vi "Dashboard Main.vi"() -> ()   [LabVIEW 2012]
uses:
  <vilib>/event_ctls.llb/eventvkey.ctl
  <vilib>/Utility/config.llb/Read Key (String).vi
  <vilib>/Utility/config.llb/Read Key (I32).vi
  <vilib>/Utility/config.llb/Write Key (String).vi
  <vilib>/Utility/config.llb/Write Key (I32).vi
  <vilib>/Utility/config.llb/NI_LVConfig.lvlib
panel:
  in  "Camera Settings":T1={"Frate Rate"=30, "Compression"=30, "Size"=1} {"Frate Rate" scale=1.0..30.0; "Size" items=["640x480", "320x240", "160x120"]}
  out "Mode":T2(ring)=enum."Auto Disabled"
  out "Camera IP":string
  in  "Dashboard Tab":T3(tab)
  out "Actual TARF Angle":dbl
  in  "Enable Autonomous":bool=TRUE
  out "Time Left":dbl
  out "Red":bool
  out "Yellow":bool
  out "Green":bool
  out "Tail Closed":bool
  in  "Climber Arm Manual":bool
  out "Climber State":dbl
  out "Actual Climber Arm Position":dbl
  out "Climber Button Unlocked":bool
  out "TARF Down":bool
  in  "Time To Lower TARF In Autonomous":u32=2100
  in  "Time Red":dbl=30.0
  in  "Time Yellow":dbl=50.0
  in  "Climber Arm Tolerance":dbl=0.5
  in  "Dump Speed Inside":dbl=5.0
  in  "Dump Speed Outside":dbl=3.0
  out "TeleOp Elapsed Seconds":dbl
  in  "Autonomous Tarf Angle":dbl=29.0
  in  "Slider":dbl(slide) scale=0.0..100.0 scale format="%#_3g"
  in  "On/Off":bool caption="Solenoid"
  in  "Test Name":u16(ring) items=["Select the test to run...", "Example Test", "-------------------------------", "List of tests is built in robot code.", "Replace with your own automated tests."]
  in  "Test Tree":string(tree)
  in  "Motor":cluster{"Value":dbl, "Enable":bool} {"Value" scale=-1.0..1.0 scale format="%#_3g"}
  out "Progress":T4 {"Test Progress" scale=0.0..100.0}
  in  "Rev/Fwd":cluster{"Forward":bool, "Reverse":bool}
  in  "Ring":u16(ring) items=["Auto", "Fixed indoor", "Fixed outdoor 1", "Fixed outdoor 2", "Fixed fluorescent 1", "Fixed fluorescent 2", "Hold current"]
  in  "Listbox":i32(listbox)
  in  "Viewer":enum32{"Camera Image", "Variables"}(tab)
  out "Mbps":dbl format="%#.1g"
  in  "Enable":bool
  in  "DB Camera Config":bool
  out "Mbps":bool
  out "fps":dbl format="%#.1g"
  out "Image Error Message":string="Timeout in Camera Communications"
  out "Camera Image":T5(plugin-control)
  out "Robot IP":string
  out "Tree":string(tree)
  # "Robot IP:"
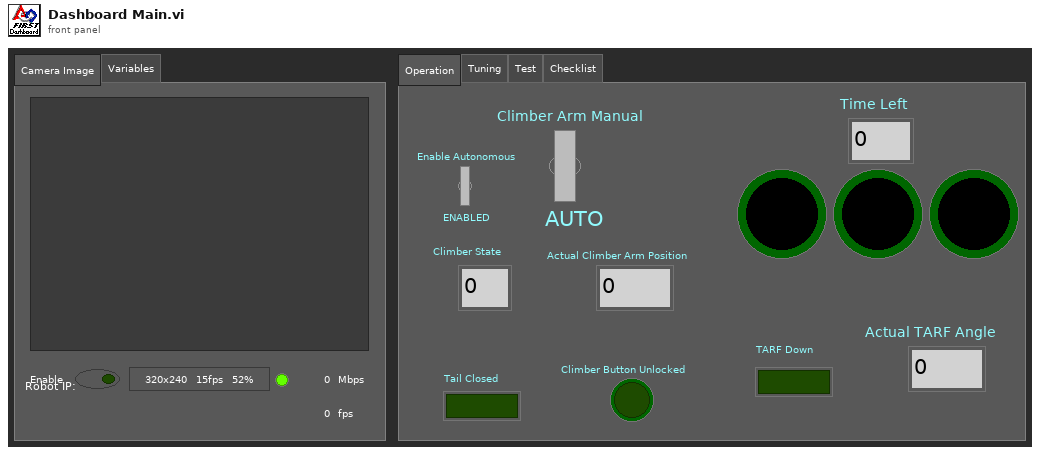
[diagram p1: front panel]
types:
  T1 = cluster{"Frate Rate":i32, "Compression":i32, "Size":u16}
  T2 = enum8{"Tele-Op Disabled", "Tele-Op Enabled", "Auto Disabled", "Auto Enabled", "Test Disabled", "Test Enabled", ""}
  T3 = enum32{"Operation", "Tuning", "Test", "Checklist"}
  T4 = cluster{"Test Progress":u8, "Test Progress Text":string}
  T5 = typedef "IMAQ Image.ctl" = refnum<image>
  T6 = typedef "Image Type" = u32
  T7 = typedef "SkeletonTrackState.ctl" = enum32{"NotTracked", "PositionOnly", "Tracked"}
  T8 = cluster{"TrackingState":u8[], "Position":cluster{"x":sgl, "y":sgl, "z":sgl}, cluster{"x":sgl, "y":sgl, "z":sgl, sgl}[], "TrackState":T7}
  T9 = cluster{cluster{"ScaledToPercentRange":dbl, "ScaledToPercentRange":dbl, "ScaledToPercentRange":dbl}, cluster{bool, bool, bool}}[]
  T10 = cluster{cluster{"ScaledToPercentRange":dbl, "ScaledToPercentRange":dbl, "ScaledToPercentRange":dbl}, cluster{bool, bool, bool}}
  T11 = typedef "LVRectTypeDef.ctl" = cluster{"Left":i16, "Top":i16, "Right":i16, "Bottom":i16}
  T12 = cluster{"Competition mode":bool, "Robot Link":bool, "Autonomous":bool, "Enabled":bool, "E-Stop":bool, "Simulated":bool, "TestMode":bool, "Docked Window":bool}
  T13 = typedef "NI_LVConfig.lvlib/Config Data RefNum.ctl" = refnum<k1>
  T14 = typedef "eventvkey.ctl" = enum16{"ASCII", "Enter", "Return", "Shift", "Ctrl", "Alt", "Cmd", "Opt", "Caps", "NumLock", "Clear", "Break", "Up", "Down", "Left", "Right", "Insert", "Delete", "Home", "End", "PageUp", "PageDown", "Escape", "Help", "Pause", "ScrollLock", "F1", "F2", "F3", "F4", "F5", "F6", "F7", "F8", "F9", "F10", "F11", "F12", "F13", "F14", "F15", "F16", "F17", "F18", "F19", "F20", "F21", "F22", "F23", "F24", "Play", "VolumeUp", "VolumeDown", "Mute", "Two Byte Char"}
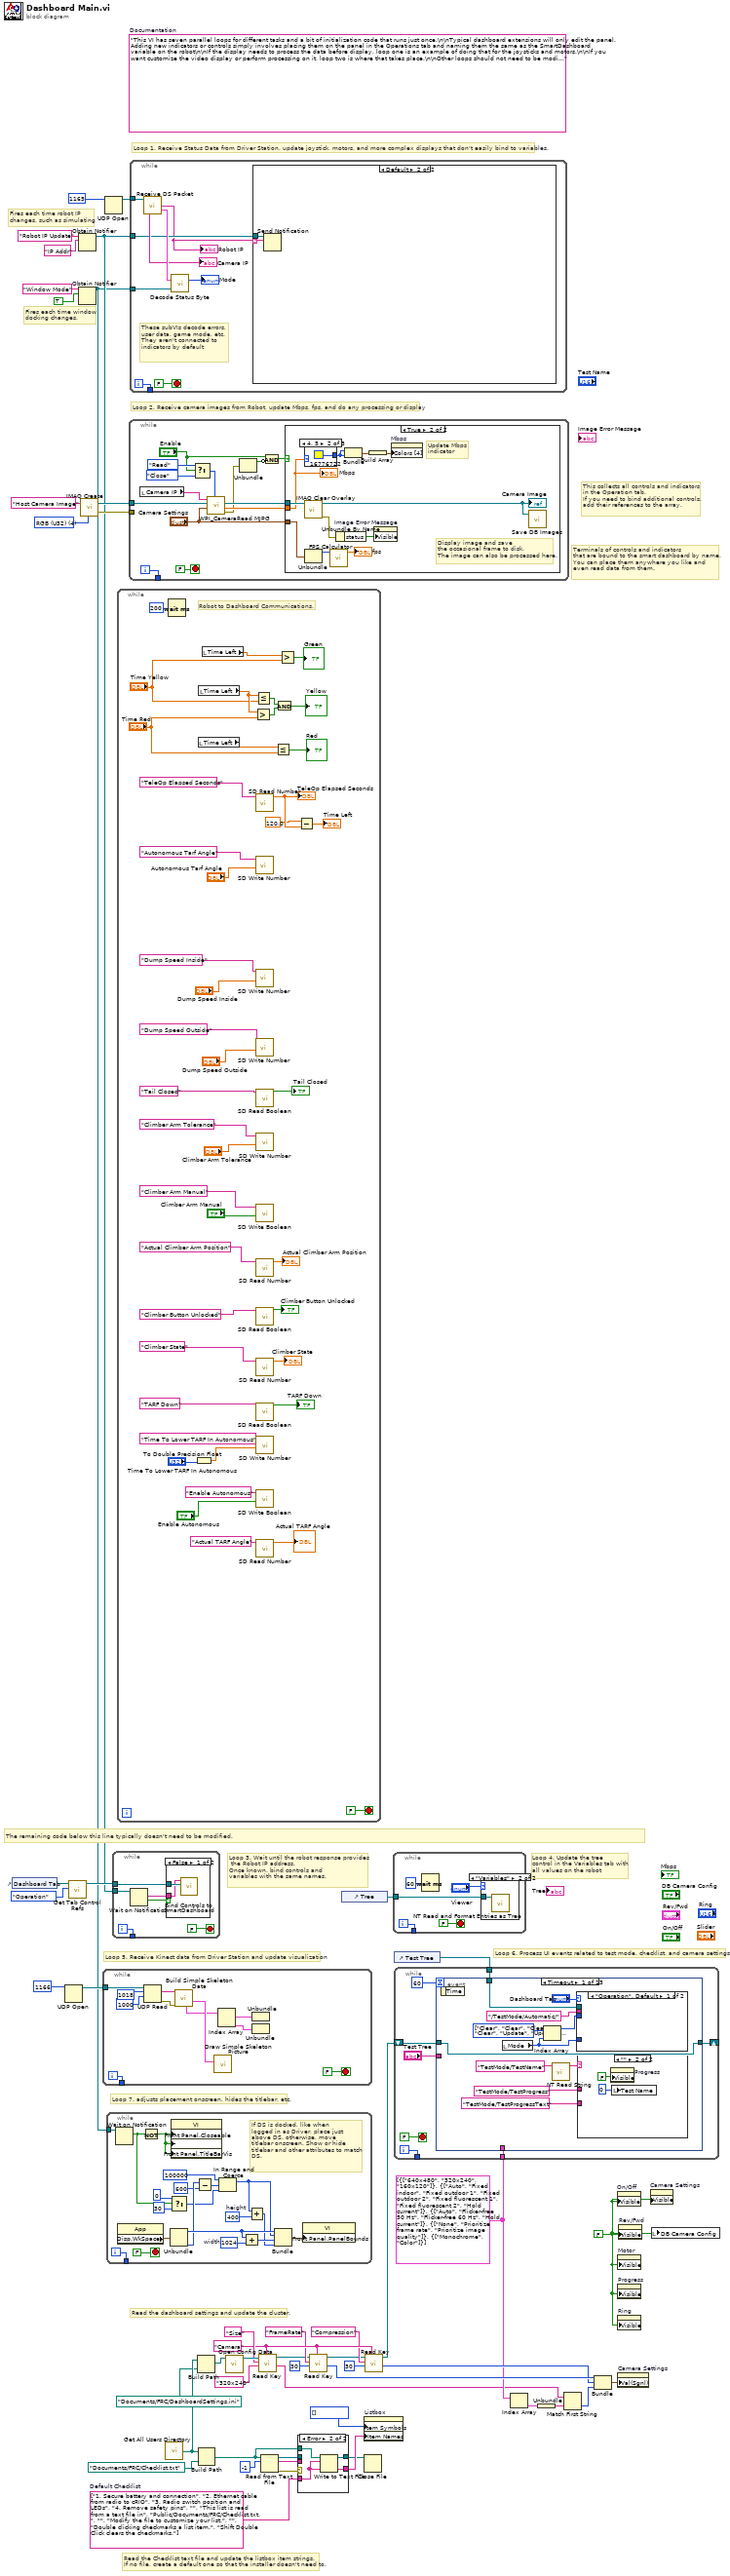
[diagram p0: block diagram]
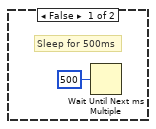
[diagram p3: hidden frame]
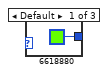
[diagram p4: hidden frame]
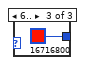
[diagram p5: hidden frame]
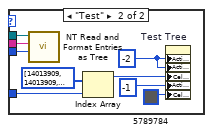
[diagram p7: hidden frame]
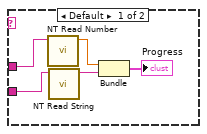
[diagram p8: hidden frame]
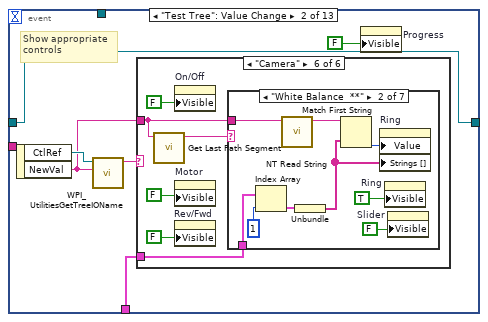
[diagram p9: hidden frame]
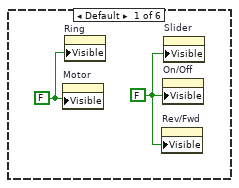
[diagram p10: hidden frame]
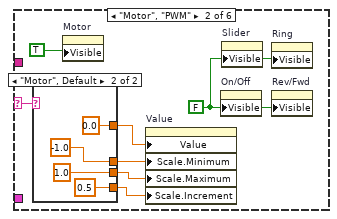
[diagram p11: hidden frame]
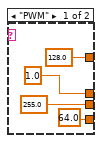
[diagram p12: hidden frame]
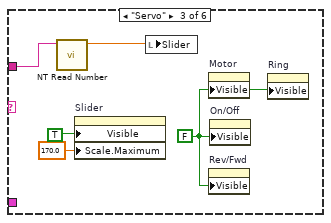
[diagram p13: hidden frame]
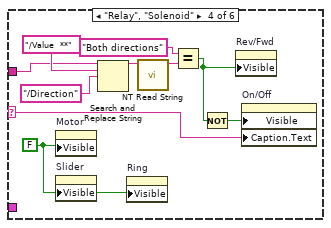
[diagram p14: hidden frame]
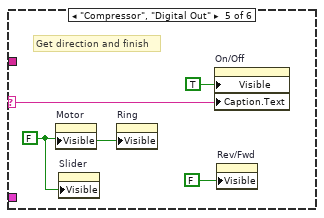
[diagram p15: hidden frame]
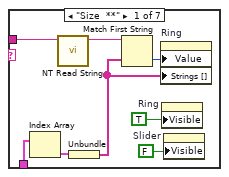
[diagram p16: hidden frame]
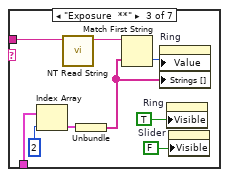
[diagram p17: hidden frame]
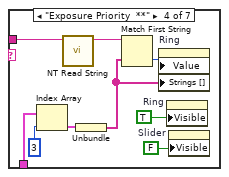
[diagram p18: hidden frame]
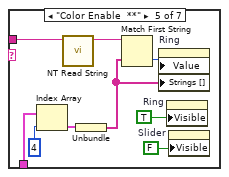
[diagram p19: hidden frame]
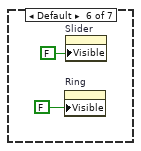
[diagram p20: hidden frame]
diagram:
  w21 = "Camera"
  w13 = cluster{string[]}[] [{["640x480", "320x240", "160x120"]}, {["Auto", "Fixed indoor", "Fixed outdoor 1", "Fixed outdoor 2", "Fixed fluorescent 1", "Fixed fluorescent 2", "Hold current"]}, {["Auto", "Flicker-free 50 Hz", "Flicker-free 60 Hz", "Hold current"]}, {["None", "Prioritize frame rate", "Prioritize image quality"]}, {["Monochrome", "Color"]}]
  w29 = string[] ["1. Secure battery and connection", "2. Ethernet cable from radio to cRIO", "3. Radio switch position and LEDs", "4. Remove safety pins", "", "This list is read from a text file in", "Public/Documents/FRC/Checklist.txt.", "", "Modify the file to customize your list.", "", "Double clicking checkmarks a list item.", "Shift Double Click clears the checkmarks."]  # Default Checklist
  w27 = FALSE ("Visible")
  (unwired) "This VI has seven parallel loops for different tasks and a bit of initialization code that runs just once.\n\nTypical dashboard extensions will only edit the panel. Adding new indicators or controls simply involves placing them on the panel in the Operations tab and naming them the same as the SmartDashboard variable on the robot\n\nIf the display needs to process the data before display, loop one is an example of doing that for the joysticks and motors.\n\nIf you want customize the video display or perform processing on it, loop two is where that takes place.\n\nOther loops should not need to be modified. They are pretty standard, and document the task they perform."  # Documentation
  w50 = T6 4 items=["Grayscale (U8)", "Grayscale (I16)", "Grayscale (SGL)", "Complex (CSG)", "RGB (U32)", "HSL (U32)", "RGB (U64)"] ("Image Type")
  # "Terminals of controls and indicators\nthat are bound to the smart dashboard by name.\nYou can place them anywhere you like and\neven read data from them."
  # "Fires each time robot IP\nchanges, such as simulating"
  # "Fires each time window\ndocking changes."
  # "Read the Checklist text file and update the listbox item strings.\nIf no file, create a default one so that the installer doesn't need to."
  # "This collects all controls and indicators\nin the Operation tab.\nIf you need to bind additional controls,\nadd their references to the array."
  # "The remaining code below this line typically doesn't need to be modified."
  # "Loop 6. Process UI events related to test mode, checklist, and camera settings"
  # "Read the dashboard settings and update the cluster."
  # "Loop 4. Update the tree\ncontrol in the Variables tab with\nall values on the robot"
  # "Loop 3. Wait until the robot response provides\n the Robot IP address.\nOnce known, bind controls and\nvariables with the same names."
  # "Loop 5. Receive Kinect data from Driver Station and update visualization"
  # "Loop 7. adjusts placement onscreen, hides the titlebar, etc."
  # "Loop 1. Receive Status Data from Driver Station, update joystick, motors, and more complex displays that don't easily bind to variables."
  # "Loop 2. Receive camera images from Robot, update Mbps, fps, and do any processing or display"
  n1 = control-ref of="Dashboard Tab"() -> (w43:refnum<vi>)
  n2 = UDP Open(11:u16 1166 ("port")) -> (port=w45:refnum<k16>)  [unwired: 2 in, 4 out]
  n3 = call <vilib>:"Get Tab Control Refs.vi"("Page Index"=enum32{"Operation", "Test"}."Operation" ("Dashboard Tab"), "TabControl in"=w43) -> ("ControlsOnPage"=w44:refnum<vi>[])  [unwired: 9 in]
  n4 = Obtain Notifier(name (unnamed)="Robot IP Update", notification data type="IP Addr" ("name (unnamed)")) -> (notifier out=w40:refnum<notifier>)  [unwired: 2 in, 2 out]
  n5 = Obtain Notifier(name (unnamed)="Window Mode", notification data type=TRUE) -> (notifier out=w33:refnum<notifier>)  [unwired: 2 in, 2 out]
  n6 = call "IMAQ Create"("Image Name"="Host Camera Image", "Image Type"=w50) -> ("New Image"=w48:T5, "error out"=w47:errorcluster)  [unwired: 2 in, 1 out]
  n7 = while {
    tunnel: w45 -> [w61]
    tunnel: [w54] -> _
    i -> [w54]
    stop <- FALSE stop-if-true
    n8 = UDP Read(connection ID=w61, max size (548)=1018 ("bytes to read"), timeout ms (25000)=1000) -> (data out=w59:string, error out=w53:errorcluster)  [unwired: 1 in, 3 out]
    n9 = call "Build Simple Skeleton Data.vi"("error in (no error)"=w53, "data in"=w59) -> ("Skeleton Data"=w60:T8, "Simple Joystick Info"=w57:T9)  [unwired: 5 in, 3 out]
    n10 = call "Draw Simple Skeleton Picture.vi"("Simple Skeleton"=w60) -> ()  [unwired: 10 in, 1 out]
    n11 = Index Array(array=w57) -> (element #1=w56:T10, element #2=w55:T10)  [unwired: 2 in]
    n12 = Unbundle(w56) -> ()  [unwired: 2 out]
    n13 = Unbundle(w55) -> ()  [unwired: 2 out]
  }
  n14 = UDP Open(11:u16 1165 ("port")) -> (port=w51:refnum<k16>)  [unwired: 2 in, 4 out]
  n15 = while {
    tunnel: w33 -> [w82]
    tunnel: [w80] -> _
    i -> [w80]
    stop <- FALSE stop-if-true
    w72 = 1024  # width
    w75 = 400  # height
    # "If DS is docked, like when\nlogged in as Driver, place just\nabove DS, otherwise, move\ntitlebar onscreen. Show or hide\ntitlebar and other attributes to match\nDS."
    n16 = Wait on Notification(notifier=w82) -> (notification=w67:bool)  [unwired: 3 in, 3 out]
    n17 = property class="App"() -> ("Disp.WkSpace"=w78:T11)  [unwired: 2 in, 2 out]
    n18 = Not(x=w67) -> (.not. x?=w81:bool)
    n19 = Unbundle(w78) -> ("Left"=w76:i16, "Bottom"=w73:i16)  [unwired: 2 out]
    n20 = Select(t=0, s=w67, f=30) -> (s? t:f=w66:i32)
    n21 = property class="VI"("Front Panel.Closeable"=w81, "Front Panel.Minimizeable"=w81, "Front Panel.TitleBarVis"=w81) -> ()  [unwired: 2 in, 2 out]
    n22 = Subtract(x=w73, y=600) -> (x-y=w70:i32)
    n23 = In Range and Coerce(upper limit=100000, x=w70, lower limit=w66) -> (coerced(x)=w64:i32)  [unwired: 1 out]
    n24 = Add(x=w76, y=w72) -> (x+y=w77:i32)
    n25 = Add(x=w64, y=w75) -> (x+y=w74:i32)
    n26 = Bundle("Left"=w76, w64, w77, w74) -> (w79:cluster{"Left":i16, i32, i32, i32})  [unwired: 1 out]
    n27 = property class="VI"("Front Panel.PanelBounds"=w79) -> ()  [unwired: 2 in, 2 out]
  }
  n28 = while {
    tunnel: w44 -> [w89]
    tunnel: w40 -> [w86]
    tunnel: [w84] -> _
    i -> [w84]
    stop <- FALSE stop-if-true
    n29 = Wait on Notification(notifier=w86) -> (notification=w85:string, timed out?=w87:bool)  [unwired: 3 in, 2 out]
    n30 = case shown="False" w87 {
      tunnel: w89 -> [w91 _]
      tunnel: w85 -> [w90 _]
      frame False {
        n31 = call <vilib>:"Bind Controls to SmartDashboard.vi"("Bound Control Refs"=w91, "Server IP Address"=w90) -> ()  [unwired: 10 in]
      }
      frame True {
      }
    }
  }
  n32 = while {
    stop <- FALSE stop-if-true
    # "Robot to Dashboard Communications."
    n33 = Wait (ms)(milliseconds to wait=u32 200) -> ()  [unwired: 1 out]
    n34 = To Double Precision Float(number="Time To Lower TARF In Autonomous") -> (double precision float=w104:dbl)
    n35 = local read "Time Left"() -> (w115:dbl)
    n36 = local read "Time Left"() -> (w119:dbl)
    n37 = local read "Time Left"() -> (w121:dbl)
    n38 = Greater?(x=w119, y="Time Red") -> (0:w117:bool)
    n39 = Less Or Equal?(x=w119, y="Time Yellow") -> (x <= y?=w118:bool)
    n40 = call <vilib>:"SD Read Number.vi"("Name"="TeleOp Elapsed Seconds") -> ("Numeric"=w112:dbl)  [unwired: 8 in, 2 out]
    "TeleOp Elapsed Seconds" <- w112
    n41 = call <vilib>:"SD Write Number.vi"("Numeric"="Autonomous Tarf Angle", "Name"="Autonomous Tarf Angle") -> ()  [unwired: 8 in, 2 out]
    n42 = call <vilib>:"SD Write Number.vi"("Numeric"="Dump Speed Inside", "Name"="Dump Speed Inside") -> ()  [unwired: 8 in, 2 out]
    n43 = call <vilib>:"SD Write Number.vi"("Numeric"="Dump Speed Outside", "Name"="Dump Speed Outside") -> ()  [unwired: 8 in, 2 out]
    n44 = call <vilib>:"SD Read Boolean.vi"("Name"="Tail Closed") -> ("Boolean"=→"Tail Closed":bool)  [unwired: 8 in, 2 out]
    n45 = call <vilib>:"SD Write Number.vi"("Numeric"="Climber Arm Tolerance", "Name"="Climber Arm Tolerance") -> ()  [unwired: 8 in, 2 out]
    n46 = call <vilib>:"SD Write Boolean.vi"("Boolean"="Climber Arm Manual", "Name"="Climber Arm Manual") -> ()  [unwired: 8 in, 2 out]
    n47 = call <vilib>:"SD Read Number.vi"("Name"="Actual Climber Arm Position") -> ("Numeric"=→"Actual Climber Arm Position":dbl)  [unwired: 8 in, 2 out]
    n48 = call <vilib>:"SD Read Boolean.vi"("Name"="Climber Button Unlocked") -> ("Boolean"=→"Climber Button Unlocked":bool)  [unwired: 8 in, 2 out]
    n49 = call <vilib>:"SD Read Number.vi"("Name"="Climber State") -> ("Numeric"=→"Climber State":dbl)  [unwired: 8 in, 2 out]
    n50 = call <vilib>:"SD Read Boolean.vi"("Name"="TARF Down") -> ("Boolean"=→"TARF Down":bool)  [unwired: 8 in, 2 out]
    n51 = call <vilib>:"SD Write Number.vi"("Numeric"=w104, "Name"="Time To Lower TARF In Autonomous") -> ()  [unwired: 8 in, 2 out]
    n52 = call <vilib>:"SD Write Boolean.vi"("Boolean"="Enable Autonomous", "Name"="Enable Autonomous") -> ()  [unwired: 8 in, 2 out]
    n53 = call <vilib>:"SD Read Number.vi"("Name"="Actual TARF Angle") -> ("Numeric"=→"Actual TARF Angle":dbl)  [unwired: 8 in, 2 out]
    n54 = Less Or Equal?(x=w115, y="Time Red") -> (x <= y?=→"Red":bool)
    n55 = And(x=w118, y=w117) -> (x .and. y?=→"Yellow":bool)
    n56 = Greater?(x=w121, y="Time Yellow") -> (0:→"Green":bool)
    n57 = Subtract(x=120.0, y=w112) -> (x-y=→"Time Left":dbl)
  }
  n58 = while {
    tunnel: w48 -> [w144]
    tunnel: w47 -> [_]
    tunnel: [w147] -> _
    i -> [w147]
    stop <- FALSE stop-if-true
    n59 = local read "Camera IP"() -> (w146:string)
    n60 = Select(t=enum16{"Read", "Reopen", "Close"}."Read" ("Operation"), s="Enable", f=enum16{"Read", "Reopen", "Close"}."Close" ("Operation")) -> (s? t:f=w139:enum16{"Read", "Reopen", "Close"})
    n61 = call <vilib>:"WPI_CameraRead MJPG.vi"("Operation"=w139, "Camera Settings"="Camera Settings", "Image"=w144, "address"=w146) -> ("error out"=w138:errorcluster, "Bandwidth (kbps)"=w142:dbl, "Image Out"=w143:T5)  [unwired: 5 in]
    n62 = Unbundle(w138) -> ("status"=w136:bool)  [unwired: 2 out]
    n63 = Compound Arithmetic op=AND("Enable", invert w136) -> (w135:bool)
    n64 = case shown="True" w135 {
      tunnel: "Camera Settings" -> [_ w151]
      tunnel: w143 -> [_ w154]
      tunnel: w142 -> [_ w153]
      frame False {
        # "Sleep for 500ms"
        n65 = Wait Until Next ms Multiple(millisecond multiple=u32 500) -> ()  [unwired: 1 out]
      }
      frame True {
        # "Display image and save\nthe occasional frame to disk.\nThe image can also be processed here."
        # "Update Mbps\nindicator"
        n66 = call "IMAQ Clear Overlay"("Image"=w154) -> ("error out"=w159:errorcluster, "Image Out"=w158:T5)  [unwired: 2 in, 7 out]
        "Camera Image" <- w158
        n67 = case shown="4, 5" w153 {
          tunnel: [u32 6618880 ("Color Box") u32 16776722 ("Color Box") u32 16716800 ("Color Box")] -> w155
          frame Default {
          }
          frame 4, 5 {
          }
          frame 6.. {
          }
        }
        n68 = Unbundle(w151) -> ("Frate Rate"=w150:i32)  [unwired: 2 out]
        n69 = call "FPS Calculator.vi"("Average Count"=w150) -> ("fps"=→"fps":dbl)  [unwired: 10 in]
        n70 = Unbundle By Name(w159) -> ("status"=w160:bool)
        n71 = Bundle("Color Box"=w155, "Color Box"=w155) -> (w157:cluster{"Color Box":u32, "Color Box":u32})  [unwired: 1 out]
        n72 = Build Array(w157) -> (w156:cluster{"Color Box":u32, "Color Box":u32}[])
        n73 = property on="Image Error Message" class="Str"("Visible"=w160) -> ()  [unwired: 2 in, 2 out]
        n74 = property on="Mbps" class="Bool (strict)"("Colors [4]"=w156) -> ()  [unwired: 2 in, 2 out]
        n75 = call "Save DB Images.vi"("Image"=w158) -> ()  [unwired: 2 in, 1 out]
        "Mbps" <- w153
      }
    }
  }
  n76 = while {
    tunnel: w51 -> [w170]
    tunnel: w40 -> [w165]
    tunnel: w33 -> [w169]
    tunnel: [w166] -> _
    i -> [w166]
    stop <- FALSE stop-if-true
    # "These subVIs decode errors, user data, game mode, etc.\nThey aren't connected to indicators by default"
    n77 = call "Receive DS Packet.vi"("Recv Socket"=w170) -> ("Robot IP Address"=w164:string, "Status"=w171:T12, "Camera IP Address"=→"Camera IP":string)  [unwired: 1 in, 11 out]
    "Robot IP" <- w164
    n78 = call "Decode Status Byte.vi"("Window Mode Notifier"=w169, "Status"=w171) -> ("Mode"=→"Mode":T2)  [unwired: 1 out]
    n79 = case shown="Default" w164 {
      selector: w164 -> [_ w173]
      tunnel: w165 -> [_ w174]
      frame "0.0.0.0" {
        # "Robot not responding, don't poll the variables"
      }
      frame Default {
        n80 = Send Notification(notification=w173, notifier=w174) -> ()  [unwired: 1 in, 2 out]
      }
    }
  }
  n81 = call "Get All Users Directory.vi"() -> ("All User Path"=w26:path)
  n82 = Build Path(base path=w26, name or relative path=path "Documents/FRC/DashboardSettings.ini") -> (appended path=w25:path)
  n83 = Build Path(base path=w26, name or relative path=path "Documents/FRC/Checklist.txt") -> (appended path=w30:path)
  n84 = call <vilib>:"Open Config Data.vi"("configuration file path"=w25) -> ("refnum"=w24:T13)  [unwired: 8 in, 2 out]
  n85 = call-poly <vilib>:"Read Key.vi"("section"=w21, "default value"="320x240", "key"="Size", "refnum"=w24) -> ("value"=w11:string, "refnum out"=w6:T13)  [unwired: 2 in, 4 out]
  n86 = Read from Text File(file (use dialog)=w30, count=-1 ("timeout ms (25000)")) -> (refnum out=w8:refnum<file>, text=w31:string[], error out=w32:errorcluster)  [unwired: 2 in, 1 out]
  n87 = case shown="Error" w32 {
    tunnel: w31 -> [w176 _]
    tunnel: [w176 w178] -> w28
    tunnel: w29 -> [_ w178]
    tunnel: w30 -> [_ w179]
    tunnel: [w175 w177] -> w7
    tunnel: w8 -> [w175 _]
    frame No Error {
    }
    frame Error {
      n88 = Write to Text File(file (use dialog)=w179, text=w178) -> (refnum out=w177:refnum<file>)  [unwired: 2 in, 2 out]
    }
  }
  n89 = call-poly <vilib>:"Read Key.vi"("section"=w21, "default value"=30, "key"="FrameRate", "refnum"=w6) -> ("value"=w16:i32, "refnum out"=w5:T13)  [unwired: 1 in, 5 out]
  n90 = control-ref of="Tree"() -> (w2:refnum<vi>)
  n91 = property on="Listbox" class="LstBox (strict)"("Item Symbols"=i32[] [], "Item Names"=w28) -> ()  [unwired: 2 in, 2 out]
  n92 = Close File(refnum=w7) -> ()  [unwired: 1 in, 2 out]
  n93 = call-poly <vilib>:"Read Key.vi"("section"=w21, "default value"=30, "key"="Compression", "refnum"=w5) -> ("value"=w15:i32, "refnum out"=w3:T13)  [unwired: 1 in, 5 out]
  n94 = while {
    tunnel: [w181] -> _
    tunnel: w2 -> [w180]
    i -> [w181]
    stop <- FALSE stop-if-true
    n95 = Wait (ms)(milliseconds to wait=u32 60) -> ()  [unwired: 1 out]
    n96 = case shown="\"Variables\"" "Viewer" {
      tunnel: w180 -> [_ w185]
      frame Default {
      }
      frame "Variables" {
        n97 = call <vilib>:"NT Read and Format Entries as Tree.vi"("Tree Refnum"=w185) -> ()  [unwired: 9 in, 2 out]
      }
    }
  }
  n98 = control-ref of="Test Tree"() -> (w1:refnum<vi>)
  n99 = while {
    tunnel: w13 -> [w190]
    shift-right: [w189] -> _
    shift-left: w3 -> [w188]
    tunnel: [w187] -> _
    tunnel: w1 -> [w186]
    i -> [w187]
    stop <- FALSE stop-if-true
    n100 = event shown="[0] Timeout" {
      selector: _ -> [_ _ _ _ _ _ _ _ _ _ _ _ _]
      dyn-events: _ -> [_ _ _ _ _ _ _ _ _ _ _ _ _]
      timeout: u32 60 ("milliseconds to wait") -> [_ _ _ _ _ _ _ _ _ _ _ _ _]
      tunnel: w186 -> [w200 _ _ _ _ _ _ _ _ _ _ _ _]
      tunnel: "Test Tree" -> [_ _ _ _ _ _ _ _ w394 w402 w404 w408 w416]
      tunnel: w190 -> [_ w222 _ _ _ _ w358 w388 _ _ _ _ _]
      tunnel: [w194 w221 _ w324 w332 w344 w357 w381 w393 w400 w403 w407 w415] -> w189
      tunnel: w188 -> [w194 w221 _ w324 w332 w344 w356 w381 w393 w400 w403 w407 w415]
      event Timeout {
        w199 = enum16{"Update", "Clear"}[] [enum."Clear", enum."Clear", enum."Clear", enum."Clear", enum."Update", enum."Update", enum."Clear"] items=["Update", "Clear"]
        n101 = event-data() -> ()  [unwired: 1 in, 1 out]
        n102 = local read "Mode"() -> (w197:T2)
        n103 = Index Array(array=w199, index=w197) -> (element=w198:enum16{"Update", "Clear"})
        n104 = call <vilib>:"NT Read String.vi"("Name"="TestMode/TestName") -> ("String"=w203:string)  [unwired: 9 in, 1 out]
        n105 = case shown="\"Operation\", Default" "Dashboard Tab" {
          tunnel: w200 -> [_ w213]
          tunnel: "/TestMode/Automatic/" ("Name Pattern") -> [_ w212]
          tunnel: w198 -> [_ w211]
          tunnel: w197 -> [_ w209]
          frame "Operation", Default {
          }
          frame "Test" {
            w208 = -2 ("Active Item:Row Number")
            n106 = call <vilib>:"NT Read and Format Entries as Tree.vi"("Operation"=w211, "Name Pattern"=w212, "Tree Refnum"=w213) -> ()  [unwired: 7 in, 2 out]
            n107 = Index Array(array=u32[] [14013909, 14013909, 14013909, 14013909, 14013909, 16777215, 14013909], index=w209) -> (element=w207:u32)
            n108 = property on="Test Tree" class="Tree (strict)"("Active Item Row Number"=w208, "ActiveColNum"=w208, "CellBG"=w207, "Active Item Row Number"=-1 ("Active Item:Row Number"), "CellBG"=u32 5789784 ("Color Box")) -> ()  [unwired: 2 in, 2 out]
          }
        }
        n109 = case shown="\"\"" w203 {
          tunnel: "TestMode/TestProgress" ("Name") -> [w215 _]
          tunnel: "TestMode/TestProgressText" ("Name") -> [w214 _]
          frame Default {
            n110 = call <vilib>:"NT Read Number.vi"("Name"=w215) -> ("Numeric"=w216:dbl)  [unwired: 9 in, 1 out]
            n111 = call <vilib>:"NT Read String.vi"("Name"=w214) -> ("String"=w217:string)  [unwired: 9 in, 1 out]
            n112 = Bundle("Numeric"=w216, "String"=w217) -> (→"Progress":cluster{"Numeric":dbl, "String":string})  [unwired: 1 in]
          }
          frame "" {
            n113 = property on="Progress" class="Clust (strict)"("Visible"=FALSE) -> ()  [unwired: 2 in, 2 out]
            n114 = local write "Test Name"(u16 0) -> ()
          }
        }
      }
      event "Test Tree": Value Change {
        # "Show appropriate\ncontrols"
        n115 = event-data() -> ("CtlRef"=w225:refnum<vi>, "NewVal"=w223:string)  [unwired: 1 in]
        n116 = call <vilib>:"WPI_UtilitiesGetTreeIOName.vi"("NewVal"=w223, "TreeControl in"=w225) -> ("I/O Name"=w226:string)  [unwired: 9 in]
        n117 = case shown="\"Camera\"" w226 {
          selector: w226 -> [_ w233 _ w251 w260 _]
          tunnel: w223 -> [_ _ w248 w250 _ w267]
          tunnel: w222 -> [_ _ _ _ _ w266]
          frame Default {
            w228 = FALSE ("Visible")
            w227 = FALSE ("Visible")
            n118 = property on="Motor" class="Clust (strict)"("Visible"=w227) -> ()  [unwired: 2 in, 2 out]
            n119 = property on="Ring" class="Ring (strict)"("Visible"=w227) -> ()  [unwired: 2 in, 2 out]
            n120 = property on="Rev/Fwd" class="Clust (strict)"("Visible"=w228) -> ()  [unwired: 2 in, 2 out]
            n121 = property on="On/Off" class="Bool (strict)"("Visible"=w228) -> ()  [unwired: 2 in, 2 out]
            n122 = property on="Slider" class="Slide (strict)"("Visible"=w228) -> ()  [unwired: 2 in, 2 out]
          }
          frame "Motor", "PWM" {
            w234 = FALSE ("Visible")
            n123 = case shown="\"Motor\", Default" w233 {
              tunnel: [1.0 ("Value") -1.0 ("Value")] -> w232
              tunnel: [255.0 ("Value") 1.0 ("Value")] -> w231
              tunnel: [128.0 ("Value") 0.0 ("Value")] -> w230
              tunnel: [64.0 ("Value") 0.5 ("Value")] -> w229
              frame "PWM" {
              }
              frame "Motor", Default {
              }
            }
            n124 = property on="Motor" class="Clust (strict)"("Visible"=TRUE) -> ()  [unwired: 2 in, 2 out]
            n125 = property on="Value" class="Slide (strict)"("Value"=w230, "Scale.Minimum"=w232, "Scale.Maximum"=w231, "Scale.Increment"=w229) -> ()  [unwired: 2 in, 2 out]
            n126 = property on="On/Off" class="Bool (strict)"("Visible"=w234) -> ()  [unwired: 2 in, 2 out]
            n127 = property on="Slider" class="Slide (strict)"("Visible"=w234) -> ()  [unwired: 2 in, 2 out]
            n128 = property on="Ring" class="Ring (strict)"("Visible"=w234) -> ()  [unwired: 2 in, 2 out]
            n129 = property on="Rev/Fwd" class="Clust (strict)"("Visible"=w234) -> ()  [unwired: 2 in, 2 out]
          }
          frame "Servo" {
            w246 = FALSE ("Visible")
            n130 = call <vilib>:"NT Read Number.vi"("Name"=w248) -> ("Numeric"=w247:dbl)  [unwired: 9 in, 1 out]
            n131 = property on="Slider" class="Slide (strict)"("Visible"=TRUE, "Scale.Maximum"=170.0 ("Scale.Range:Maximum")) -> ()  [unwired: 2 in, 2 out]
            n132 = local write "Slider"(w247) -> ()
            n133 = property on="Motor" class="Clust (strict)"("Visible"=w246) -> ()  [unwired: 2 in, 2 out]
            n134 = property on="Rev/Fwd" class="Clust (strict)"("Visible"=w246) -> ()  [unwired: 2 in, 2 out]
            n135 = property on="On/Off" class="Bool (strict)"("Visible"=w246) -> ()  [unwired: 2 in, 2 out]
            n136 = property on="Ring" class="Ring (strict)"("Visible"=w246) -> ()  [unwired: 2 in, 2 out]
          }
          frame "Relay", "Solenoid" {
            w249 = FALSE ("Visible")
            n137 = property on="Motor" class="Clust (strict)"("Visible"=w249) -> ()  [unwired: 2 in, 2 out]
            n138 = property on="Slider" class="Slide (strict)"("Visible"=w249) -> ()  [unwired: 2 in, 2 out]
            n139 = Search and Replace String(input string=w250, search string="/Value  **", replace string="/Direction") -> (result string=w256:string)  [unwired: 5 in, 3 out]
            n140 = property on="Ring" class="Ring (strict)"("Visible"=w249) -> ()  [unwired: 2 in, 2 out]
            n141 = call <vilib>:"NT Read String.vi"("Name"=w256) -> ("String"=w254:string)  [unwired: 9 in, 1 out]
            n142 = Equal?(x="Both directions", y=w254) -> (x = y?=w252:bool)
            n143 = Not(x=w252) -> (.not. x?=w253:bool)
            n144 = property on="Rev/Fwd" class="Clust (strict)"("Visible"=w252) -> ()  [unwired: 2 in, 2 out]
            n145 = property on="On/Off" class="Bool (strict)"("Visible"=w253, "Caption.Text"=w251) -> ()  [unwired: 2 in, 2 out]
          }
          frame "Compressor", "Digital Out" {
            w259 = FALSE ("Visible")
            # "Get direction and finish"
            n146 = property on="Motor" class="Clust (strict)"("Visible"=w259) -> ()  [unwired: 2 in, 2 out]
            n147 = property on="Slider" class="Slide (strict)"("Visible"=w259) -> ()  [unwired: 2 in, 2 out]
            n148 = property on="Ring" class="Ring (strict)"("Visible"=w259) -> ()  [unwired: 2 in, 2 out]
            n149 = property on="On/Off" class="Bool (strict)"("Visible"=TRUE, "Caption.Text"=w260) -> ()  [unwired: 2 in, 2 out]
            n150 = property on="Rev/Fwd" class="Clust (strict)"("Visible"=FALSE) -> ()  [unwired: 2 in, 2 out]
          }
          frame "Camera" {
            n151 = call <vilib>:"Get Last Path Segment.vi"("String in"=w267) -> ("String out"=w268:string)  [unwired: 10 in]
            n152 = property on="On/Off" class="Bool (strict)"("Visible"=FALSE) -> ()  [unwired: 2 in, 2 out]
            n153 = property on="Motor" class="Clust (strict)"("Visible"=FALSE) -> ()  [unwired: 2 in, 2 out]
            n154 = property on="Rev/Fwd" class="Clust (strict)"("Visible"=FALSE) -> ()  [unwired: 2 in, 2 out]
            n155 = case shown="\"White Balance  **\"" w268 {
              tunnel: w267 -> [w274 w283 w292 w301 w310 _ w316]
              tunnel: w266 -> [w272 w280 w289 w298 w307 _ _]
              frame "Size  **" {
                n156 = Index Array(array=w272) -> (element=w271:cluster{string[]})  [unwired: 1 in]
                n157 = call <vilib>:"NT Read String.vi"("Name"=w274) -> ("String"=w273:string)  [unwired: 9 in, 1 out]
                n158 = Unbundle(w271) -> (w269:string[])
                n159 = Match First String(2:w269, 3:w273) -> (0:w270:i32)  [unwired: 1 out]
                n160 = property on="Ring" class="Ring (strict)"("Value"=w270, "Strings []"=w269) -> ()  [unwired: 2 in, 2 out]
                n161 = property on="Ring" class="Ring (strict)"("Visible"=TRUE) -> ()  [unwired: 2 in, 2 out]
                n162 = property on="Slider" class="Slide (strict)"("Visible"=FALSE) -> ()  [unwired: 2 in, 2 out]
              }
              frame "White Balance  **" {
                n163 = Index Array(array=w280, index=1) -> (element=w281:cluster{string[]})
                n164 = call <vilib>:"NT Read String.vi"("Name"=w283) -> ("String"=w282:string)  [unwired: 9 in, 1 out]
                n165 = Unbundle(w281) -> (w278:string[])
                n166 = Match First String(2:w278, 3:w282) -> (0:w277:i32)  [unwired: 1 out]
                n167 = property on="Ring" class="Ring (strict)"("Value"=w277, "Strings []"=w278) -> ()  [unwired: 2 in, 2 out]
                n168 = property on="Ring" class="Ring (strict)"("Visible"=TRUE) -> ()  [unwired: 2 in, 2 out]
                n169 = property on="Slider" class="Slide (strict)"("Visible"=FALSE) -> ()  [unwired: 2 in, 2 out]
              }
              frame "Exposure  **" {
                n170 = Index Array(array=w289, index=2) -> (element=w290:cluster{string[]})
                n171 = call <vilib>:"NT Read String.vi"("Name"=w292) -> ("String"=w291:string)  [unwired: 9 in, 1 out]
                n172 = Unbundle(w290) -> (w286:string[])
                n173 = Match First String(2:w286, 3:w291) -> (0:w287:i32)  [unwired: 1 out]
                n174 = property on="Ring" class="Ring (strict)"("Value"=w287, "Strings []"=w286) -> ()  [unwired: 2 in, 2 out]
                n175 = property on="Ring" class="Ring (strict)"("Visible"=TRUE) -> ()  [unwired: 2 in, 2 out]
                n176 = property on="Slider" class="Slide (strict)"("Visible"=FALSE) -> ()  [unwired: 2 in, 2 out]
              }
              frame "Exposure Priority  **" {
                n177 = Index Array(array=w298, index=3) -> (element=w299:cluster{string[]})
                n178 = call <vilib>:"NT Read String.vi"("Name"=w301) -> ("String"=w300:string)  [unwired: 9 in, 1 out]
                n179 = Unbundle(w299) -> (w295:string[])
                n180 = Match First String(2:w295, 3:w300) -> (0:w296:i32)  [unwired: 1 out]
                n181 = property on="Ring" class="Ring (strict)"("Value"=w296, "Strings []"=w295) -> ()  [unwired: 2 in, 2 out]
                n182 = property on="Ring" class="Ring (strict)"("Visible"=TRUE) -> ()  [unwired: 2 in, 2 out]
                n183 = property on="Slider" class="Slide (strict)"("Visible"=FALSE) -> ()  [unwired: 2 in, 2 out]
              }
              frame "Color Enable  **" {
                n184 = Index Array(array=w307, index=4) -> (element=w308:cluster{string[]})
                n185 = call <vilib>:"NT Read String.vi"("Name"=w310) -> ("String"=w309:string)  [unwired: 9 in, 1 out]
                n186 = Unbundle(w308) -> (w304:string[])
                n187 = Match First String(2:w304, 3:w309) -> (0:w305:i32)  [unwired: 1 out]
                n188 = property on="Ring" class="Ring (strict)"("Value"=w305, "Strings []"=w304) -> ()  [unwired: 2 in, 2 out]
                n189 = property on="Ring" class="Ring (strict)"("Visible"=TRUE) -> ()  [unwired: 2 in, 2 out]
                n190 = property on="Slider" class="Slide (strict)"("Visible"=FALSE) -> ()  [unwired: 2 in, 2 out]
              }
              frame Default {
                n191 = property on="Ring" class="Ring (strict)"("Visible"=FALSE) -> ()  [unwired: 2 in, 2 out]
                n192 = property on="Slider" class="Slide (strict)"("Visible"=FALSE) -> ()  [unwired: 2 in, 2 out]
              }
              frame "Brightness  **", "Color Level  **", "Compression  **", "FPS  **", "Sharpness  **" {
                n193 = call <vilib>:"NT Read Number.vi"("Name"=w316) -> ("Numeric"=w315:dbl)  [unwired: 9 in, 1 out]
                n194 = local write "Slider"(w315) -> ()
                n195 = property on="Slider" class="Slide (strict)"("Visible"=TRUE, "Scale.Maximum"=100.0 ("Scale.Range:Maximum")) -> ()  [unwired: 2 in, 2 out]
                n196 = property on="Ring" class="Ring (strict)"("Visible"=FALSE) -> ()  [unwired: 2 in, 2 out]
              }
            }
          }
        }
        n197 = property on="Progress" class="Clust (strict)"("Visible"=FALSE) -> ()  [unwired: 2 in, 2 out]
      }
      event "Test Name": Mouse Enter {
        # "Populate the ring with the list of tests"
        n198 = event-data() -> ()  [unwired: 1 in, 1 out]
        n199 = call <vilib>:"NT Read String Array.vi"("Name"="TestMode/TestList") -> ("String Array"=w323:string[])  [unwired: 9 in, 1 out]
        n200 = Build Array (concatenate)("Select the test to run...", w323) -> (w322:string[])
        n201 = property on="Test Name" class="Ring (strict)"("Strings []"=w322) -> ()  [unwired: 2 in, 2 out]
      }
      event "Test Name": Value Change {
        w325 = FALSE ("Visible")
        # "Tell the robot the test name to run"
        n202 = event-data() -> ("NewVal"=w329:u16)  [unwired: 1 in]
        n203 = property on="Test Name" class="Ring (strict)"() -> ("Strings []"=w330:string[])  [unwired: 2 in, 2 out]
        n204 = local write "Progress"(T4 {"Test Progress"=0, "Test Progress Text"=""} ("Progress")) -> ()
        n205 = Index Array(array=w330, index=w329) -> (element=w328:string)
        n206 = call <vilib>:"NT Write String.vi"("String"=w328, "Name"="TestMode/TestName") -> ()  [unwired: 9 in, 1 out]
        n207 = property on="Progress" class="Clust (strict)"("Visible"=TRUE) -> ()  [unwired: 2 in, 2 out]
        n208 = property on="Motor" class="Clust (strict)"("Visible"=w325) -> ()  [unwired: 2 in, 2 out]
        n209 = property on="Slider" class="Slide (strict)"("Visible"=w325) -> ()  [unwired: 2 in, 2 out]
        n210 = property on="On/Off" class="Bool (strict)"("Visible"=w325) -> ()  [unwired: 2 in, 2 out]
        n211 = property on="Rev/Fwd" class="Clust (strict)"("Visible"=w325) -> ()  [unwired: 2 in, 2 out]
        n212 = property on="Ring" class="Ring (strict)"("Visible"=w325) -> ()  [unwired: 2 in, 2 out]
      }
      event "Listbox": Double Click {
        n213 = event-data() -> ("PlatMods.Shift"=w333:bool, "Row"=w335:i32)  [unwired: 1 in]
        n214 = case shown="False" w333 {
          tunnel: w335 -> [w339 _]
          tunnel: 1 -> [w338 _]
          frame False {
            n215 = property on="Listbox" class="LstBox (strict)"() -> ("Item Symbols"=w337:i32[])  [unwired: 2 in, 2 out]
            n216 = Replace Array Subset(array=w337, new element=w338, index=w339) -> (w336:i32[])
            n217 = property on="Listbox" class="LstBox (strict)"("Item Symbols"=w336) -> ()  [unwired: 2 in, 2 out]
          }
          frame True {
            w340 = 0 ("Top Row")
            n218 = property on="Listbox" class="LstBox (strict)"() -> ("Number of Rows"=w342:u32)  [unwired: 2 in, 2 out]
            n219 = Initialize Array(0, w342) -> (w341:i32[])
            n220 = property on="Listbox" class="LstBox (strict)"("Top Row"=w340, "Value"=w340, "Item Symbols"=w341) -> ()  [unwired: 2 in, 2 out]
          }
        }
      }
      event "Listbox": Key Down {
        n221 = event-data() -> ("VKey"=w346:T14)  [unwired: 1 in]
        n222 = case shown="\"Left\", \"Right\"" w346 {
          selector: w346 -> [w351 _]
          tunnel: eventvkey."Left" ("VKey") -> [w349 _]
          frame "Left", "Right" {
            n223 = Equal?(x=w349, y=w351) -> (x = y?=w350:bool)
            n224 = Select(t=0, s=w350, f=1) -> (s? t:f=w352:i32)
            n225 = property on="Listbox" class="LstBox (strict)"() -> ("Item Symbols"=w355:i32[])  [unwired: 2 in, 2 out]
            n226 = Replace Array Subset(array=w355, new element=w352, index="Listbox") -> (w354:i32[])
            n227 = property on="Listbox" class="LstBox (strict)"("Item Symbols"=w354) -> ()  [unwired: 2 in, 2 out]
          }
          frame Default {
          }
        }
      }
      event "DB Camera Config": Value Change {
        n228 = event-data() -> ("NewVal"=w359:bool)  [unwired: 1 in]
        n229 = case shown="False" w359 {
          tunnel: w358 -> [w368 _]
          tunnel: [w361 w379] -> w357
          tunnel: w356 -> [w360 w379]
          frame False {
            w375 = "Camera"
            w378 = FALSE ("Visible")
            n230 = local read "Camera Settings"() -> (w367:T1)
            n231 = Index Array(array=w368) -> (element=w371:cluster{string[]})  [unwired: 1 in]
            n232 = Unbundle(w367) -> ("Frate Rate"=w366:i32, "Compression"=w365:i32, "Size"=w369:u16)
            n233 = Unbundle(w371) -> (w370:string[])
            n234 = Index Array(array=w370, index=w369) -> (element=w364:string)
            n235 = call-poly <vilib>:"Write Key.vi"("section"=w375, "value"=w364, "key"="Size", "refnum"=w360) -> ("refnum out"=w377:T13)  [unwired: 2 in, 5 out]
            n236 = call-poly <vilib>:"Write Key.vi"("section"=w375, "value"=w366, "key"="FrameRate", "refnum"=w377) -> ("refnum out"=w376:T13)  [unwired: 1 in, 6 out]
            n237 = property on="Camera Settings" class="Clust (strict)"("Visible"=w378) -> ()  [unwired: 2 in, 2 out]
            n238 = local write "DB Camera Config"(w378) -> ()
            n239 = call-poly <vilib>:"Write Key.vi"("section"=w375, "value"=w365, "key"="Compression", "refnum"=w376) -> ("refnum out"=w362:T13)  [unwired: 1 in, 6 out]
            n240 = call <vilib>:"Close Config Data.vi"("refnum"=w362) -> ("file path"=w363:path)  [unwired: 2 in, 8 out]
            n241 = call <vilib>:"Open Config Data.vi"("configuration file path"=w363) -> ("refnum"=w361:T13)  [unwired: 8 in, 2 out]
          }
          frame True {
            n242 = property on="Camera Settings" class="Clust (strict)"("Visible"=TRUE) -> ()  [unwired: 2 in, 2 out]
          }
        }
      }
      event "Camera Settings": Value Change {
        n243 = event-data() -> ("NewVal"=w392:T1)  [unwired: 1 in]
        n244 = Index Array(array=w388) -> (element=w387:cluster{string[]})  [unwired: 1 in]
        n245 = Unbundle(w392) -> ("Frate Rate"=w383:i32, "Compression"=w382:i32, "Size"=w385:u16)
        n246 = Unbundle(w387) -> (w386:string[])
        n247 = Index Array(array=w386, index=w385) -> (element=w384:string)
        n248 = Format Into String(format string="%s   %dfps   %d%%", w384, w383, w382) -> (resulting string=w389:string)  [unwired: 2 in, 1 out]
        n249 = Build Array(w389) -> (w390:string[])
        n250 = property on="DB Camera Config" class="Bool (strict)"("Strings [4]"=w390) -> ()  [unwired: 2 in, 2 out]
      }
      event "Motor.Enable": Value Change {
        n251 = event-data() -> ("NewVal"=w398:bool)  [unwired: 1 in]
        n252 = Unbundle("Motor") -> ("Value"=w397:dbl)  [unwired: 1 out]
        n253 = Select(t=w397, s=w398, f=0.0) -> (s? t:f=w395:dbl)
        n254 = call <vilib>:"NT Write Number.vi"("Numeric"=w395, "Name"=w394) -> ()  [unwired: 9 in, 1 out]
      }
      event "Slider": Value Change {
        n255 = event-data() -> ("NewVal"=w401:dbl)  [unwired: 1 in]
        n256 = call <vilib>:"NT Write Number.vi"("Numeric"=w401, "Name"=w402) -> ()  [unwired: 9 in, 1 out]
      }
      event "On/Off": Value Change {
        n257 = event-data() -> ("NewVal"=w406:bool)  [unwired: 1 in]
        n258 = Boolean To (0,1)(Boolean=w406) -> (0, 1=w405:i16)
        n259 = call <vilib>:"NT Write Number.vi"("Numeric"=w405, "Name"=w404) -> ()  [unwired: 9 in, 1 out]
      }
      event "Rev/Fwd": Value Change {
        n260 = event-data() -> ("NewVal.Forward"=w414:bool, "NewVal.Reverse"=w413:bool)  [unwired: 1 in]
        n261 = Boolean To (0,1)(Boolean=w414) -> (0, 1=w410:i16)
        n262 = Boolean To (0,1)(Boolean=w413) -> (0, 1=w412:i16)
        n263 = Negate(x=w412) -> (-x=w411:i16)
        n264 = Add(x=w410, y=w411) -> (x+y=w409:i16)
        n265 = call <vilib>:"NT Write Number.vi"("Numeric"=w409, "Name"=w408) -> ()  [unwired: 9 in, 1 out]
      }
      event "Ring": Value Change {
        n266 = event-data() -> ("NewVal"=w418:u16)  [unwired: 1 in]
        n267 = property on="Ring" class="Ring (strict)"() -> ("Strings []"=w419:string[])  [unwired: 2 in, 2 out]
        n268 = Index Array(array=w419, index=w418) -> (element=w417:string)
        n269 = call <vilib>:"NT Write String.vi"("String"=w417, "Name"=w416) -> ()  [unwired: 9 in, 1 out]
      }
    }
  }
  n270 = Index Array(array=w13) -> (element=w14:cluster{string[]})  [unwired: 1 in]
  n271 = Unbundle(w14) -> (w12:string[])
  n272 = Match First String(2:w12, 3:w11) -> (0:w10:i32)  [unwired: 1 out]
  n273 = Bundle("value"=w16, "value"=w15, "index"=w10) -> (w4:cluster{"value":i32, "value":i32, "index":i32})  [unwired: 1 out]
  n274 = property on="On/Off" class="Bool (strict)"("Visible"=w27) -> ()  [unwired: 2 in, 2 out]
  n275 = property on="Motor" class="Clust (strict)"("Visible"=w27) -> ()  [unwired: 2 in, 2 out]
  n276 = property on="Progress" class="Clust (strict)"("Visible"=w27) -> ()  [unwired: 2 in, 2 out]
  n277 = property on="Ring" class="Ring (strict)"("Visible"=w27) -> ()  [unwired: 2 in, 2 out]
  n278 = property on="Camera Settings" class="Clust (strict)"("Val(Sgnl)"=w4) -> ()  [unwired: 2 in, 2 out]
  n279 = property on="Rev/Fwd" class="Clust (strict)"("Visible"=w27) -> ()  [unwired: 2 in, 2 out]
  n280 = property on="Camera Settings" class="Clust (strict)"("Visible"=w27) -> ()  [unwired: 2 in, 2 out]
  n281 = local write "DB Camera Config"(w27) -> ()
